vi "Periodic Tasks.vi"(8 "error in":errorcluster) -> ()   [LabVIEW 2015]
doc: "This VI runs in parallel to other tasks. It can contain as many user-defined periodic loops as you need. These can carry out PID or other sorts of timed response."
uses:
  <vilib>/Rock Robotics/WPI/Utilities/WPI_GetSetVariantRefNum.vi
  <vilib>/Rock Robotics/Network Tables/NT Read Boolean.vi
  <vilib>/Rock Robotics/Network Tables/NT Write Number.vi
  GyroPlaceHolder.vi
  GyroLastValue.vi
  <vilib>/Rock Robotics/SystemInterfaces/Encoder/FPGA_EncoderIdx.ctl
  <vilib>/Rock Robotics/SystemInterfaces/Counter/FPGA_CounterCtrSystemIndex.ctl
  <vilib>/Rock Robotics/WPI/Encoder/WPI_EncoderType.ctl
  <vilib>/Rock Robotics/WPI/Encoder/WPI_EncoderDevRef.ctl
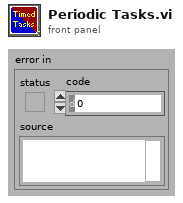
[diagram p1: front panel]
types:
  T1 = typedef "WPI_JoystickDevRef.ctl" = cluster{"Device":T2}
  T2 = typedef "WPI_JoystickDeviceEnum.ctl" = enum16{"USB 0", "USB 1", "USB 2", "USB 3", "USB 4", "USB 5"}
  T3 = typedef "WPI_RobotDriveDevRef.ctl" = cluster{"DevStatus":errorcluster, "Motors[]":T4[], "Square Inputs":bool, "Max Output":dbl}
  T4 = typedef "WPI_MotorControlDeviceRef.ctl" = cluster{"DeviceStatus":errorcluster, "Type":T5, "PWM":cluster{"PWM Channel":T6, "DeadBand":T7}, "CAN":cluster{"Device Number":u8, "Control Mode":T8, "Semaphore":T9, "Max Vout":dbl, "TalonSRX Control Mode":T10}, "Invert":bool}
  T5 = typedef "WPI_MotorControlType.ctl" = enum16{"PWM", "CAN", "CANTalonSRX"}
  T6 = typedef "FPGA_DIOPWMChannel.ctl" = enum8{"PWM 0", "PWM 1", "PWM 2", "PWM 3", "PWM 4", "PWM 5", "PWM 6", "PWM 7", "PWM 8", "PWM 9", "PWM MXP 0", "PWM MXP 1", "PWM MXP 2", "PWM MXP 3", "PWM MXP 4", "PWM MXP 5", "PWM MXP 6", "PWM MXP 7", "PWM MXP 8", "PWM MXP 9", "Invalid"}
  T7 = typedef "WPI_PWMDeadband.ctl" = cluster{"Name":string, "maxPositivePwm":i32, "minPositivePwm":i32, "centerPwm":i32, "maxNegativePwm":i32, "minNegativePwm":i32, "angularRange":u16}
  T8 = typedef "WPI_CANJaguar_ControlMode.ctl" = enum8{"Percent VBus", "Current", "Speed", "Position", "Voltage"}
  T9 = typedef "Semaphore RefNum" = refnum<k1>
  T10 = typedef "WPI_CANTalonSRX_APIControlMode.ctl" = enum8{"Percent VBus", "Speed", "Position", "Slave", "Unchanged / Invalid", "Voltage Compensation", "Current", "Motion Profile"}
  T11 = cluster{"JoystickDevRef":T1, "RobotDriveDevRef":T3}
  T12 = typedef "WPI_EncoderDevRef.ctl" = cluster{"DevStatus":errorcluster, "EncoderIndex":T13, "CounterIndex":T14, "DistancePerCount":dbl, "Decoding Type":T15}
  T13 = typedef "FPGA_EncoderIdx.ctl" = enum8{"Enc 0", "Enc 1", "Enc 2", "Enc 3", "Enc 4", "Enc 5", "Enc 6", "Enc 7", "Invalid"}
  T14 = typedef "FPGA_CounterCtrSystemIndex.ctl" = enum8{"Ctr 0", "Ctr 1", "Ctr 2", "Ctr 3", "Ctr 4", "Ctr 5", "Ctr 6", "Ctr 7", "Invalid"}
  T15 = typedef "WPI_EncoderType.ctl" = enum16{"1x", "2x", "4x"}
  T16 = typedef "WPI_AccelerometerDevRef.ctl" = cluster{"DevStatus":errorcluster, "Scaling":T17, "Analog Channels":T18, "I2C Bus":T20, "SPI Bus":T21, "Accel Range":T22, "ADXL Axes":T23, "Handle":i32, "Device Address":u8, "Accel Type":enum16{"Analog", "ADXL345 I2C", "ADXL345 SPI", "Internal", "ADXL362 SPI"}}
  T17 = typedef "WPI_AccelerometerScaling.ctl" = cluster{"Gain (VoltsPerG)":dbl, "Center Voltage":dbl}
  T18 = typedef "WPI_AccelerometerAnalogChannels.ctl" = cluster{"X-Axis":T19, "Y-Axis":T19, "Z-Axis":T19}
  T19 = typedef "FPGA_AIChannel.ctl" = enum8{"AI 0", "AI 1", "AI 2", "AI 3", "AI MXP 0", "AI MXP 1", "AI MXP 2", "AI MXP 3", "Invalid"}
  T20 = typedef "i2c_bus.ctl" = enum16{"I2C On-Board", "I2C MXP", "Invalid"}
  T21 = typedef "spi_bus.ctl" = enum16{"SPI On-Board, CS0", "SPI On-Board, CS1", "SPI On-Board, CS2", "SPI On-Board, CS3", "SPI MXP", "Invalid"}
  T22 = typedef "ADXL345 Range.ctl" = u8
  T23 = typedef "WPI_AccelerometerADXL345 Axes.ctl" = cluster{"X-Axis":bool, "Y-Axis":bool, "Z-Axis":bool}
  T24 = cluster{"X-Axis":dbl, "Y-Axis":dbl, "Z-Axis":dbl}
  T25 = typedef "WPI_GyroDevRef.ctl" = cluster{"DevStatus":errorcluster, "Analog Channel":T19, "Offset":dbl, "Gain (VoltsPerDegree/Second)":dbl, "Gyro Type":enum16{"Analog", "XRS450"}, "Handle":i32, "SPI Bus":T21, "Device Found":bool, "Sample Rate":dbl, "Calibrate On Open":bool}
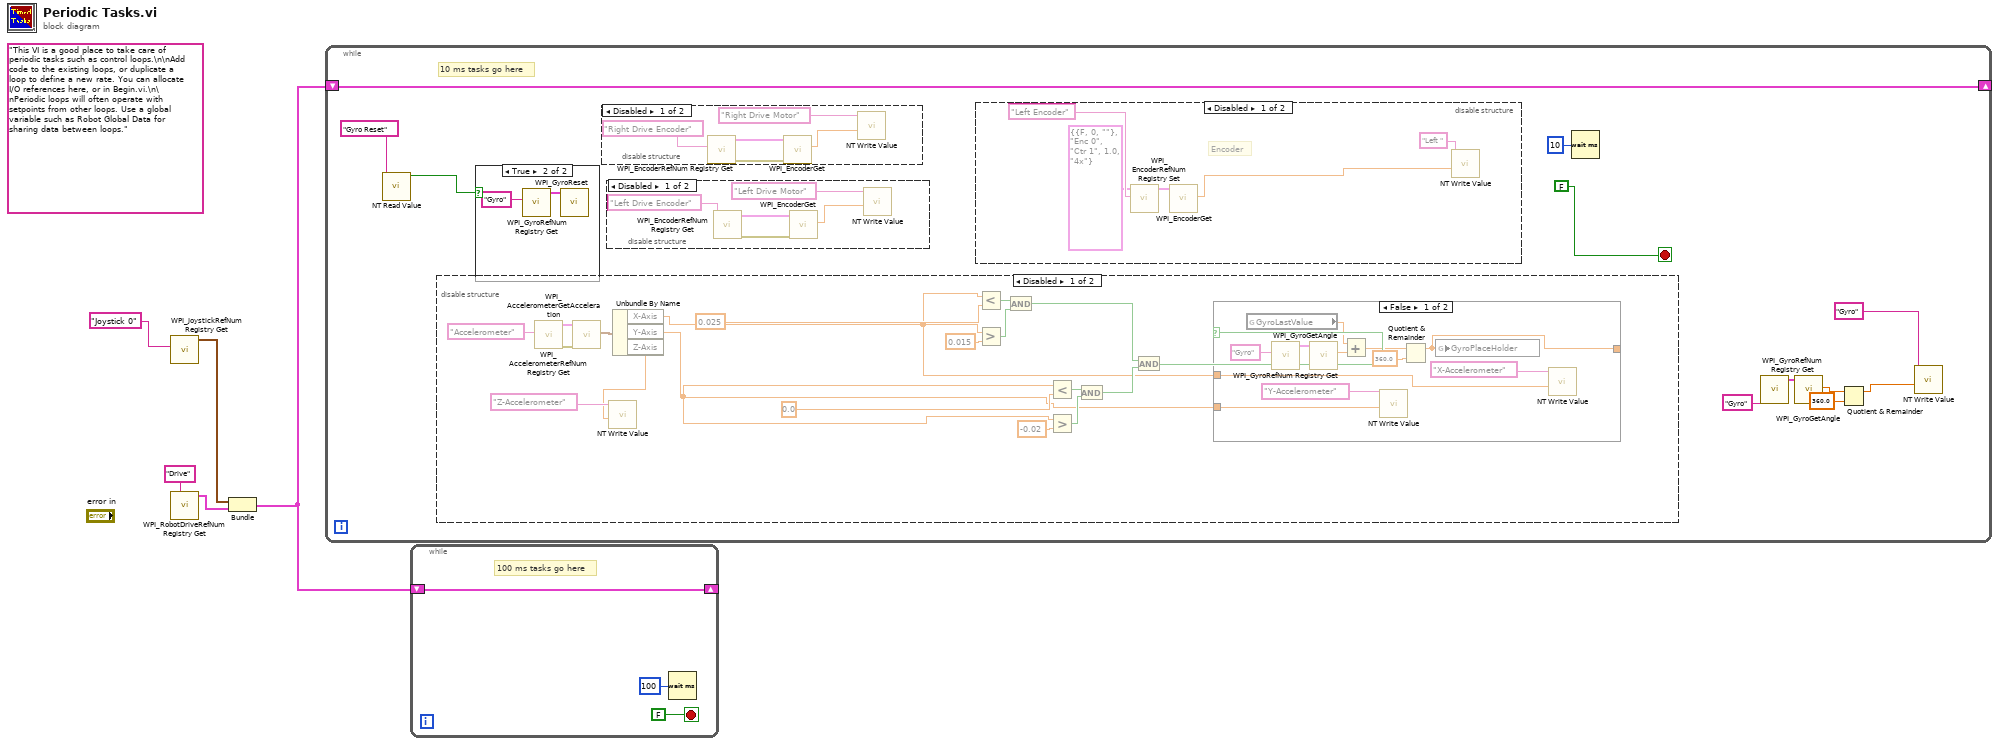
[diagram p0: block diagram]
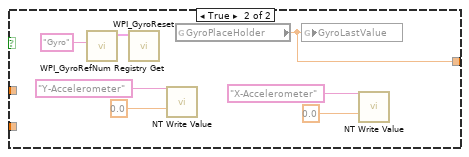
[diagram p6: hidden frame]
diagram:
  (unwired) "This VI is a good place to take care of periodic tasks such as control loops.\n\nAdd code to the existing loops, or duplicate a loop to define a new rate. You can allocate I/O references here, or in Begin.vi.\n\nPeriodic loops will often operate with setpoints from other loops. Use a global variable such as Robot Global Data for sharing data between loops."
  n1 = call <vilib>:"WPI_JoystickRefNum Registry Get.vi"("refnum name"="Joystick 0") -> ("JoystickDevRef"=w2:T1)  [unwired: 1 in, 9 out]
  n2 = call <vilib>:"WPI_RobotDriveRefNum Registry Get.vi"("refnum name"="Drive") -> ("RobotDriveDevRef"=w4:T3)  [unwired: 1 in, 9 out]
  n3 = Bundle("JoystickDevRef"=w2, "RobotDriveDevRef"=w4) -> (w1:T11)  [unwired: 1 out]
  n4 = while {
    shift-right: [w16] -> _
    shift-left: w1 -> [w16]
    stop <- FALSE stop-if-true
    # "10 ms tasks go here"
    n5 = call-poly <vilib>:"NT Read Value.vi"("Name"="Gyro Reset") -> ("Boolean"=w9:bool)  [unwired: 9 in, 1 out]
    n6 = disable-structure shown="Disabled" {
      frame Disabled {
        n7 = call <vilib>:"WPI_AccelerometerRefNum Registry Get.vi"("refnum name"="Accelerometer") -> ("error out"=w50:errorcluster, "AccelerometerDevRef"=w51:T16)  [unwired: 9 in]
        n8 = call <vilib>:"WPI_AccelerometerGetAcceleration.vi"("error in"=w50, "AccelerometerDevRef"=w51) -> ("Accelerations"=w49:T24)  [unwired: 7 in, 2 out]
        n9 = Unbundle By Name(w49) -> ("X-Axis"=w35:dbl, "Y-Axis"=w34:dbl, "Z-Axis"=w43:dbl)
        n10 = call-poly <vilib>:"NT Write Value.vi"("Numeric"=w43, "Name"="Z-Accelerometer") -> ()  [unwired: 9 in, 1 out]
        n11 = Less?(x=w35, y=0.025) -> (x < y?=w45:bool)
        n12 = Greater?(x=w35, y=0.015) -> (0:w46:bool)
        n13 = And(x=w45, y=w46) -> (x .and. y?=w37:bool)
        n14 = Less?(x=w34, y=0.0) -> (x < y?=w39:bool)
        n15 = Greater?(x=w34, y=-0.02) -> (0:w40:bool)
        n16 = And(x=w39, y=w40) -> (x .and. y?=w38:bool)
        n17 = And(x=w37, y=w38) -> (x .and. y?=w36:bool)
        n18 = case shown="False" w36 {
          tunnel: [w57 w68] -> _
          tunnel: w35 -> [w54 _]
          tunnel: w34 -> [w53 _]
          frame False {
            n19 = global read "GyroLastValue.vi" "GyroLastValue"() -> (w61:dbl)
            n20 = call <vilib>:"WPI_GyroRefNum Registry Get.vi"("refnum name"="Gyro") -> ("GyroDevRef"=w62:T25)  [unwired: 9 in, 1 out]
            n21 = call <vilib>:"WPI_GyroGetAngle.vi"("GyroDevRef"=w62) -> ("Angle"=w60:dbl)  [unwired: 6 in, 4 out]
            n22 = Add(x=w61, y=w60) -> (x+y=w58:dbl)
            n23 = call-poly <vilib>:"NT Write Value.vi"("Numeric"=w53, "Name"="Y-Accelerometer") -> ()  [unwired: 9 in, 1 out]
            n24 = Quotient & Remainder(x=w58, y=360.0) -> (x-y*floor(x/y)=w57:dbl)  [unwired: 1 out]
            n25 = global write "GyroPlaceHolder.vi" "GyroPlaceHolder"(w57) -> ()
            n26 = call-poly <vilib>:"NT Write Value.vi"("Numeric"=w54, "Name"="X-Accelerometer") -> ()  [unwired: 9 in, 1 out]
          }
          frame True {
            n27 = call <vilib>:"WPI_GyroRefNum Registry Get.vi"("refnum name"="Gyro") -> ("GyroDevRef"=w69:T25)  [unwired: 9 in, 1 out]
            n28 = call <vilib>:"WPI_GyroReset.vi"("GyroDevRef"=w69) -> ()  [unwired: 9 in, 2 out]
            n29 = call-poly <vilib>:"NT Write Value.vi"("Numeric"=0.0, "Name"="Y-Accelerometer") -> ()  [unwired: 9 in, 1 out]
            n30 = global read "GyroPlaceHolder.vi" "GyroPlaceHolder"() -> (w68:dbl)
            n31 = global write "GyroLastValue.vi" "GyroLastValue"(w68) -> ()
            n32 = call-poly <vilib>:"NT Write Value.vi"("Numeric"=0.0, "Name"="X-Accelerometer") -> ()  [unwired: 9 in, 1 out]
          }
        }
      }
      frame Enabled {
      }
    }
    n33 = case shown="True" w9 {
      frame False {
      }
      frame True {
        n34 = call <vilib>:"WPI_GyroRefNum Registry Get.vi"("refnum name"="Gyro") -> ("GyroDevRef"=w33:T25)  [unwired: 9 in, 1 out]
        n35 = call <vilib>:"WPI_GyroReset.vi"("GyroDevRef"=w33) -> ()  [unwired: 9 in, 2 out]
      }
    }
    n36 = disable-structure shown="Disabled" {
      frame Disabled {
        n37 = call <vilib>:"WPI_EncoderRefNum Registry Get.vi"("refnum name"="Right Drive Encoder") -> ("error out"=w21:errorcluster, "EncoderDevRef"=w20:T12)  [unwired: 9 in]
        n38 = call <vilib>:"WPI_EncoderGet.vi"("error in (no error)"=w21, "EncoderDevRef"=w20) -> ("Distance"=w18:dbl)  [unwired: 4 in, 5 out]
        n39 = call-poly <vilib>:"NT Write Value.vi"("Numeric"=w18, "Name"="Right Drive Motor") -> ()  [unwired: 9 in, 1 out]
      }
      frame Enabled {
      }
    }
    n40 = disable-structure shown="Disabled" {
      frame Disabled {
        n41 = call <vilib>:"WPI_EncoderRefNum Registry Get.vi"("refnum name"="Left Drive Encoder") -> ("error out"=w26:errorcluster, "EncoderDevRef"=w25:T12)  [unwired: 9 in]
        n42 = call <vilib>:"WPI_EncoderGet.vi"("error in (no error)"=w26, "EncoderDevRef"=w25) -> ("Distance"=w23:dbl)  [unwired: 4 in, 5 out]
        n43 = call-poly <vilib>:"NT Write Value.vi"("Numeric"=w23, "Name"="Left Drive Motor") -> ()  [unwired: 9 in, 1 out]
      }
      frame Enabled {
      }
    }
    n44 = disable-structure shown="Disabled" {
      frame Disabled {
        # "Encoder"
        n45 = call <vilib>:"WPI_EncoderRefNum Registry Set.vi"("refnum name"="Left Encoder", "EncoderDevRef"=T12 {"DevStatus"={"status"=FALSE, "code"=0, "source"=""}, "EncoderIndex"=enum."Enc 0", "CounterIndex"=enum."Ctr 1", "DistancePerCount"=1.0, "Decoding Type"=enum."4x"}) -> ("EncoderDevRef"=w30:T12)  [unwired: 8 in, 1 out]
        n46 = call <vilib>:"WPI_EncoderGet.vi"("EncoderDevRef"=w30) -> ("Distance"=w29:dbl)  [unwired: 5 in, 5 out]
        n47 = call-poly <vilib>:"NT Write Value.vi"("Numeric"=w29, "Name"="Left ") -> ()  [unwired: 9 in, 1 out]
      }
      frame Enabled {
      }
    }
    n48 = Wait (ms)(milliseconds to wait=u32 10) -> ()  [unwired: 1 out]
    n49 = call <vilib>:"WPI_GyroRefNum Registry Get.vi"("refnum name"="Gyro") -> ("GyroDevRef"=w12:T25)  [unwired: 9 in, 1 out]
    n50 = call <vilib>:"WPI_GyroGetAngle.vi"("GyroDevRef"=w12) -> ("Angle"=w8:dbl)  [unwired: 6 in, 4 out]
    n51 = Quotient & Remainder(x=w8, y=360.0) -> (x-y*floor(x/y)=w6:dbl)  [unwired: 1 out]
    n52 = call-poly <vilib>:"NT Write Value.vi"("Numeric"=w6, "Name"="Gyro") -> ()  [unwired: 9 in, 1 out]
  }
  n53 = while {
    shift-right: [w71] -> _
    shift-left: w1 -> [w71]
    stop <- FALSE stop-if-true
    # "100 ms tasks go here"
    n54 = Wait (ms)(milliseconds to wait=u32 100) -> ()  [unwired: 1 out]
  }
